vi "main initializer.vi"(2 "Current Baud Rate (115200)":T1=115200 items=["2400 baud"=2400, "9600 baud"=9600, "19200 baud"=19200, "38400 baud"=38400, "115200 baud"=115200], 3 "timeout (10sec)":u32=10000, 4 "VISA resource name in":refnum<visa-resource-name>="ASRL1::INSTR") -> (0 "error out":errorcluster, 1 "VISA resource name out":refnum<visa-resource-name>)   [LabVIEW 2018]
uses:
  package/controls/Sabertooth Baud Rate Select.ctl
  <vilib>/Instr/_visa.llb/VISA Configure Serial Port (Instr).vi
panel:
  # "This is the main initializer VI for the sabertooth packetized\ncontrol package. It simply wraps the init VI and UART init VI."
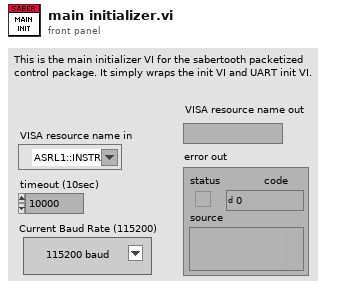
[diagram p1: front panel]
types:
  T1 = typedef "Sabertooth Baud Rate Select.ctl" = u32
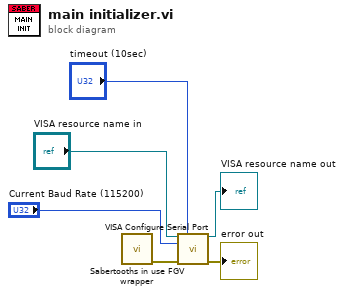
[diagram p0: block diagram]
diagram:
  n1 = call "Sabertooths in use FGV wrapper.vi"() -> ("error out"=w4:errorcluster)  [unwired: 11 in]
  n2 = call-poly "VISA Configure Serial Port"("VISA resource name"="VISA resource name in", "timeout (10sec)"="timeout (10sec)", "baud rate (9600)"="Current Baud Rate (115200)", "error in (no error)"=w4) -> ("VISA resource name out"=→"VISA resource name out":refnum<visa-resource-name>, "error out"=→"error out":errorcluster)  [unwired: 10 in]
